vi "Withdraw.vi"(8 "error in (no error)":errorcluster, 10 "Amount":dbl, 11 "ACreditAccount in":refnum<class "ACreditAccount.lvclass">) -> (0 "error out":errorcluster, 1 "Success?":bool, 2 "Balance":dbl, 3 "ACreditAccount out":refnum<class "ACreditAccount.lvclass">)   [LabVIEW 2020, in "ACreditAccount.lvclass"]
uses:
  ACreditAccount.lvclass
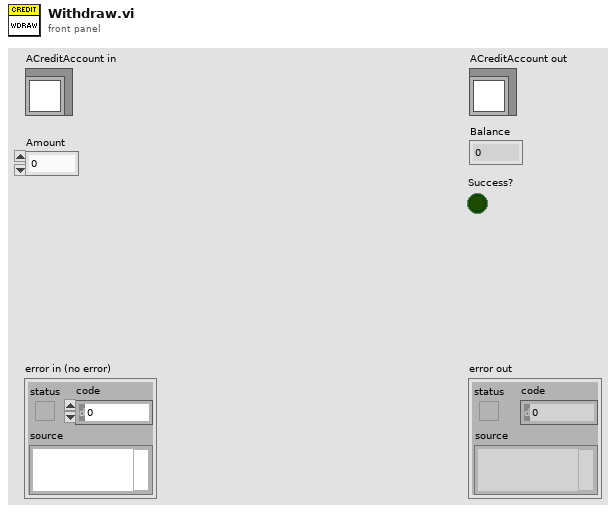
[diagram p1: front panel]
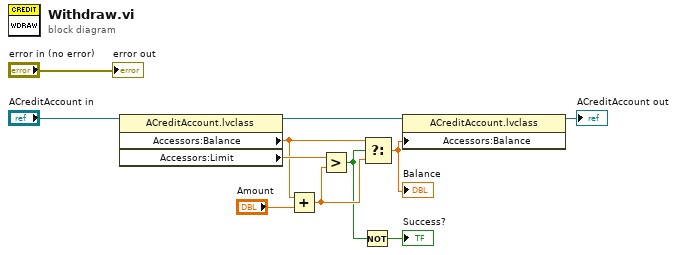
[diagram p0: block diagram]
diagram:
  n1 = property class="ACreditAccount.lvclass"(reference="ACreditAccount in") -> (reference out=w3:refnum<class "ACreditAccount.lvclass">, "Accessors:Balance"=w4:dbl, "Accessors:Limit"=w5:dbl)  [unwired: 1 in, 1 out]
  n2 = Add(x=w4, y="Amount") -> (x+y=w7:dbl)
  n3 = Greater?(x=w5, y=w7) -> (0:w6:bool)
  n4 = Not(x=w6) -> (.not. x?=→"Success?":bool)
  n5 = Select(t=w4, s=w6, f=w7) -> (s? t:f=w2:dbl)
  "Balance" <- w2
  n6 = property class="ACreditAccount.lvclass"(reference=w3, "Accessors:Balance"=w2) -> (reference out=→"ACreditAccount out":refnum<class "ACreditAccount.lvclass">)  [unwired: 1 in, 1 out]
  "error out" <- "error in (no error)"
